vi "EncoderForward.vi"(8 "EncoderDevRef 4":T2={"DevStatus"={"status"=FALSE, "code"=0, "source"=""}, "EncoderIndex"=enum."Invalid", "CounterIndex"=enum."Ctr 1", "DistancePerCount"=2.0, "Decoding Type"=enum."4x"}, 9 "RobotDriveDevRef":T6={"DevStatus"={"status"=FALSE, "code"=0, "source"=""}, "Motors[]"=[], "Square Inputs"=FALSE, "Max Output"=1.0, "Isochronous"=FALSE}, 10 "EncoderDevRef":T2={"DevStatus"={"status"=FALSE, "code"=0, "source"=""}, "EncoderIndex"=enum."Invalid", "CounterIndex"=enum."Ctr 1", "DistancePerCount"=2.0, "Decoding Type"=enum."4x"}, 11 "Target":dbl format="%#_13g") -> (0 "EncoderDevRef 3":T2={"DevStatus"={"status"=FALSE, "code"=0, "source"=""}, "EncoderIndex"=enum."Invalid", "CounterIndex"=enum."Ctr 1", "DistancePerCount"=2.0, "Decoding Type"=enum."4x"}, 1 "RobotDriveDevRef 2":T6={"DevStatus"={"status"=FALSE, "code"=0, "source"=""}, "Motors[]"=[], "Square Inputs"=FALSE, "Max Output"=1.0, "Isochronous"=FALSE}, 2 "EncoderDevRef 2":T2={"DevStatus"={"status"=FALSE, "code"=0, "source"=""}, "EncoderIndex"=enum."Invalid", "CounterIndex"=enum."Ctr 1", "DistancePerCount"=2.0, "Decoding Type"=enum."4x"})   [LabVIEW 2013]
uses:
  <vilib>/Rock Robotics/WPI/RobotDrive/WPI_RobotDriveDevRef.ctl
  <vilib>/Rock Robotics/WPI/MotorControl/WPI_MotorControlDeviceRef.ctl
  <vilib>/Rock Robotics/SystemInterfaces/Typedef/FPGA_TypedefDigitalModule.ctl
  <vilib>/Rock Robotics/SystemInterfaces/DIO/FPGA_DIOPWMChannel.ctl
  <vilib>/Rock Robotics/WPI/PWM/WPI_PWMDeadband.ctl
  <vilib>/Rock Robotics/WPI/CAN/Jaguar/SubVIs/WPI_CANJaguar_ControlMode.ctl
  <vilib>/Rock Robotics/WPI/PWM/WPI_PWMTransform_ConPane.ctl
  <vilib>/Rock Robotics/WPI/Encoder/WPI_EncoderDevRef.ctl
  <vilib>/Rock Robotics/SystemInterfaces/Encoder/FPGA_EncoderIdx.ctl
  <vilib>/Rock Robotics/SystemInterfaces/Counter/FPGA_CounterCtrSystemIndex.ctl
  <vilib>/Rock Robotics/WPI/Encoder/WPI_EncoderType.ctl
  <vilib>/addons/control/pid/pid.llb/PID (DBL).vi
  <vilib>/addons/control/pid/NI_PID_pid.lvlib
panel:
  out "dt out (s)":dbl format="%.3f"
  out "Right Distance":dbl(graph)
  out "Right Motor Power":dbl(graph)
  out "Left Motor Power":dbl(graph)
  out "Left Distance":dbl(graph)
  in  "PID gains 3":T1={"proportional gain (Kc)"=0.15, "integral time (Ti, min)"=0.0, "derivative time (Td, min)"=0.0}
  in  "output range 3":cluster{"output high":dbl, "output low":dbl}={"output high"=1.0, "output low"=-1.0}
  in  "output range 2":cluster{"output high":dbl, "output low":dbl}={"output high"=1.0, "output low"=-1.0}
  in  "PID gains 2":T1={"proportional gain (Kc)"=0.15, "integral time (Ti, min)"=0.0, "derivative time (Td, min)"=0.0}
  # "Stop?"
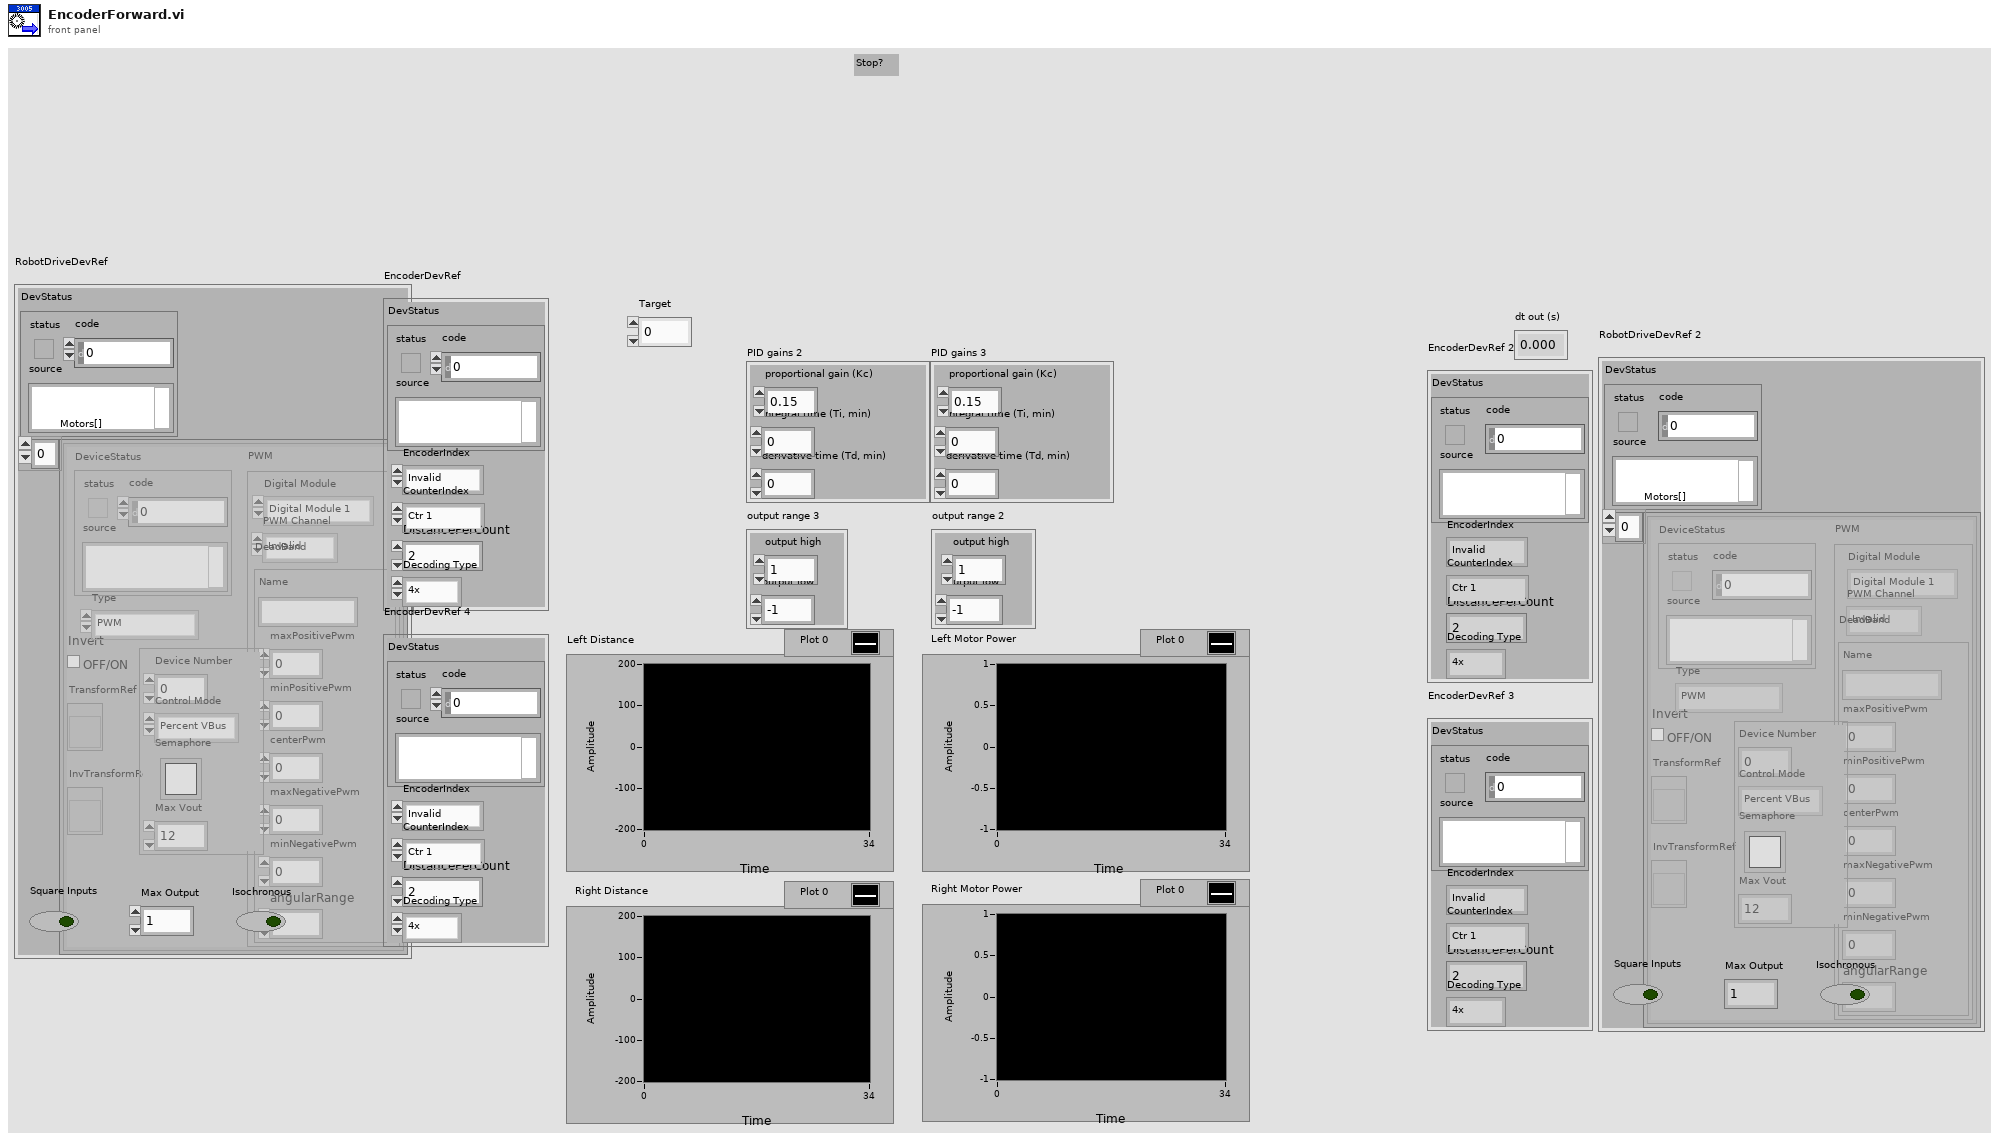
[diagram p1: front panel]
types:
  T1 = cluster{"proportional gain (Kc)":dbl, "integral time (Ti, min)":dbl, "derivative time (Td, min)":dbl}
  T2 = typedef "WPI_EncoderDevRef.ctl" = cluster{"DevStatus":errorcluster, "EncoderIndex":T3, "CounterIndex":T4, "DistancePerCount":dbl, "Decoding Type":T5}
  T3 = typedef "FPGA_EncoderIdx.ctl" = enum8{"Enc 0", "Enc 1", "Enc 2", "Enc 3", "Invalid"}
  T4 = typedef "FPGA_CounterCtrSystemIndex.ctl" = enum8{"Ctr 0", "Ctr 1", "Ctr 2", "Ctr 3", "Ctr 4", "Ctr 5", "Ctr 6", "Ctr 7", "Invalid"}
  T5 = typedef "WPI_EncoderType.ctl" = enum16{"1x", "2x", "4x"}
  T6 = typedef "WPI_RobotDriveDevRef.ctl" = cluster{"DevStatus":errorcluster, "Motors[]":T7[], "Square Inputs":bool, "Max Output":dbl, "Isochronous":bool}
  T7 = typedef "WPI_MotorControlDeviceRef.ctl" = cluster{"DeviceStatus":errorcluster, "Type":enum16{"PWM", "CAN"}, "PWM":cluster{"Digital Module":T8, "PWM Channel":T9, "DeadBand":T10}, "CAN":cluster{"Device Number":u8, "Control Mode":T11, "Semaphore":T12, "Max Vout":dbl}, "Invert":bool, "TransformRef":T13, "InvTransformRef":T13}
  T8 = typedef "FPGA_TypedefDigitalModule.ctl" = enum16{"Digital Module 1", "Digital Module 2"}
  T9 = typedef "FPGA_DIOPWMChannel.ctl" = enum8{"PWM 1", "PWM 2", "PWM 3", "PWM 4", "PWM 5", "PWM 6", "PWM 7", "PWM 8", "PWM 9", "PWM 10", "Invalid"}
  T10 = typedef "WPI_PWMDeadband.ctl" = cluster{"Name":string, "maxPositivePwm":i32, "minPositivePwm":i32, "centerPwm":i32, "maxNegativePwm":i32, "minNegativePwm":i32, "angularRange":u16}
  T11 = typedef "WPI_CANJaguar_ControlMode.ctl" = enum8{"Percent VBus", "Current", "Speed", "Position", "Voltage"}
  T12 = typedef "Semaphore RefNum" = refnum<k1>
  T13 = typedef "WPI_PWMTransform_ConPane.ctl" = refnum<vi>
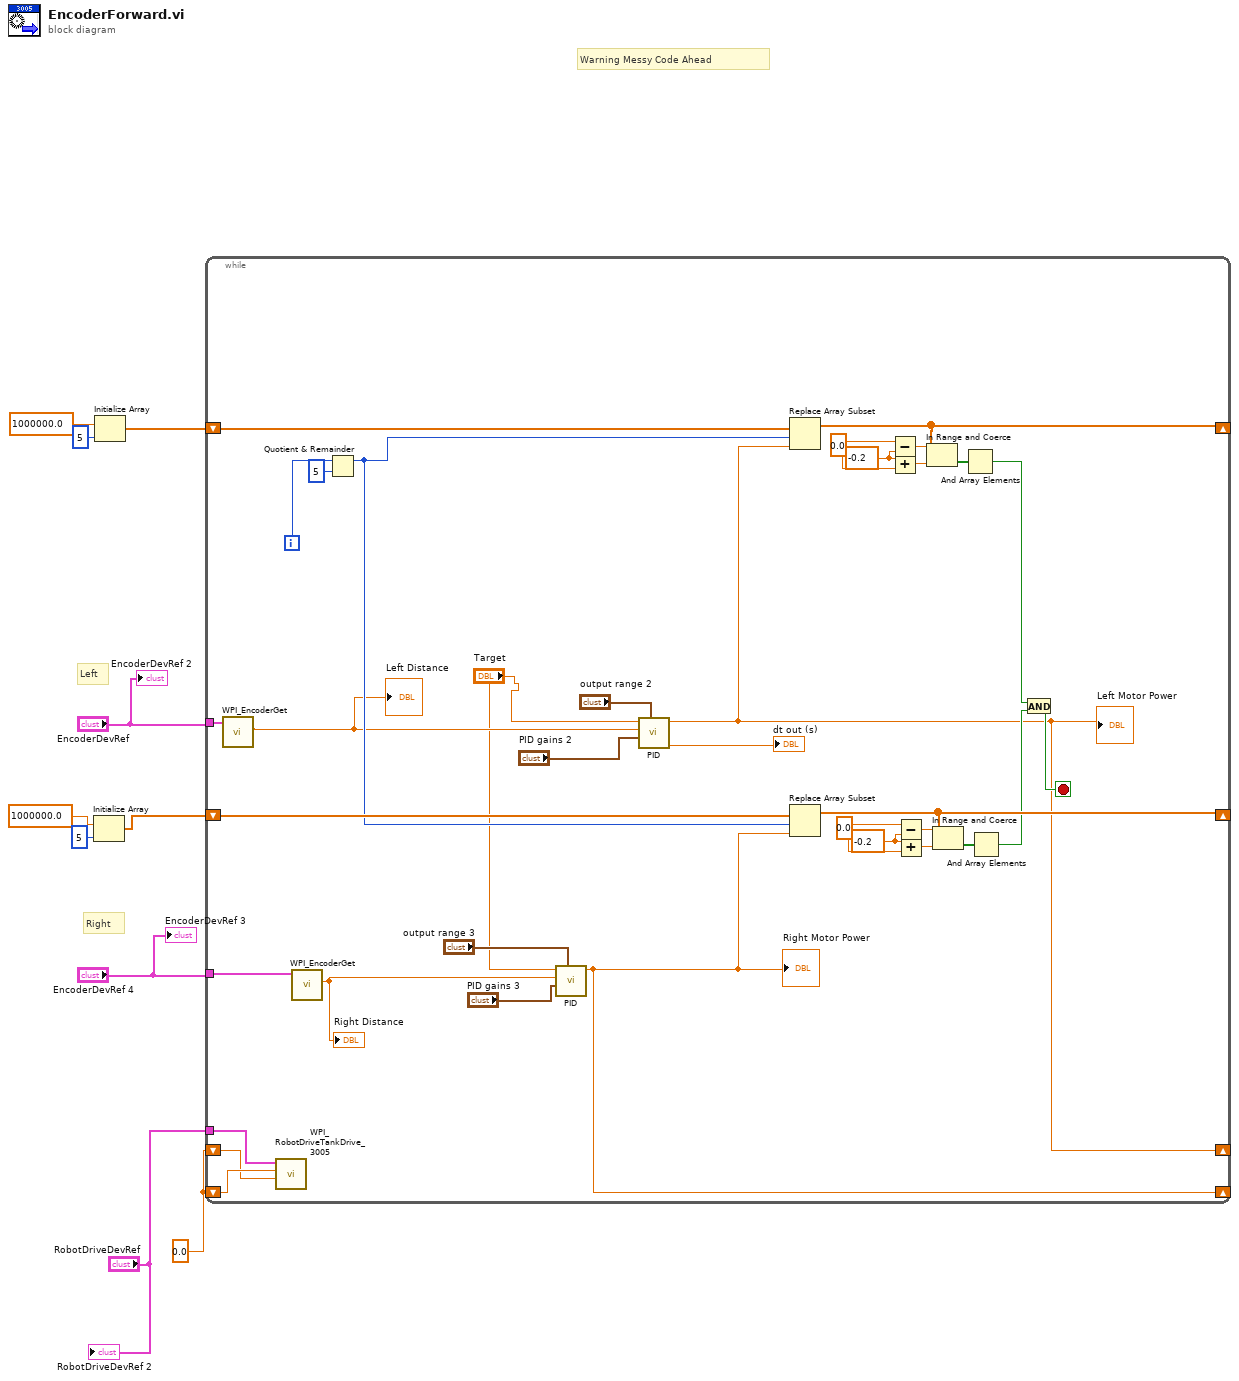
[diagram p0: block diagram]
diagram:
  w3 = 0.0 ("output")
  # "Warning Messy Code Ahead"
  # "Right"
  # "Left"
  n1 = Initialize Array(1000000.0 ("element"), 5 ("dimension size")) -> (w6:dbl[])
  n2 = Initialize Array(1000000.0 ("element"), 5 ("dimension size")) -> (w7:dbl[])
  n3 = while {
    shift-right: [w18] -> _
    shift-left: w3 -> [w28]
    tunnel: "RobotDriveDevRef" -> [w44]
    shift-right: [w12] -> _
    shift-left: w7 -> [w42]
    tunnel: "EncoderDevRef" -> [w40]
    shift-right: [w37] -> _
    shift-left: w6 -> [w34]
    tunnel: "EncoderDevRef 4" -> [w39]
    shift-right: [w21] -> _
    shift-left: w3 -> [w29]
    i -> [w41]
    stop <- w32 stop-if-true
    w13 = -0.2 ("x")
    w14 = 0.0 ("x")
    w19 = -0.2 ("x")
    w20 = 0.0 ("x")
    n4 = call <vilib>:"WPI_EncoderGet.vi"("EncoderDevRef"=w40) -> ("Distance"=w25:dbl)  [unwired: 1 in, 9 out]
    "Left Distance" <- w25
    n5 = call <vilib>:"WPI_RobotDriveTankDrive_3005.vi"("Right axis value"=w28, "Left axis value"=w29, "RobotDriveDevRef"=w44) -> ()  [unwired: 6 in, 3 out]
    n6 = call <vilib>:"WPI_EncoderGet.vi"("EncoderDevRef"=w39) -> ("Distance"=w26:dbl)  [unwired: 1 in, 9 out]
    "Right Distance" <- w26
    n7 = Quotient & Remainder(x=w41, y=5) -> (x-y*floor(x/y)=w30:i32)  [unwired: 1 out]
    n8 = call-poly <vilib>:"PID.vi"("output range"="output range 3", "PID gains"="PID gains 3", "process variable"=w26, "setpoint"="Target") -> ("output"=w21:dbl)  [unwired: 6 in, 1 out]
    "Right Motor Power" <- w21
    n9 = call-poly <vilib>:"PID.vi"("output range"="output range 2", "PID gains"="PID gains 2", "process variable"=w25, "setpoint"="Target") -> ("dt out (s)"=→"dt out (s)":dbl, "output"=w18:dbl)  [unwired: 6 in]
    "Left Motor Power" <- w18
    n10 = Replace Array Subset(array=w42, new element=w18, index=w30) -> (w12:dbl[])
    n11 = Replace Array Subset(array=w34, new element=w21, index=w30) -> (w37:dbl[])
    n12 = Subtract(x=w14, y=w13) -> (x-y=w15:dbl)
    n13 = Add(x=w13, y=w14) -> (x+y=w17:dbl)
    n14 = Subtract(x=w20, y=w19) -> (x-y=w35:dbl)
    n15 = Add(x=w19, y=w20) -> (x+y=w38:dbl)
    n16 = In Range and Coerce(upper limit=w15, x=w12, lower limit=w17) -> (In Range?=w16:bool[])  [unwired: 1 out]
    n17 = In Range and Coerce(upper limit=w35, x=w37, lower limit=w38) -> (In Range?=w36:bool[])  [unwired: 1 out]
    n18 = And Array Elements(Boolean array=w16) -> (logical AND=w11:bool)
    n19 = And Array Elements(Boolean array=w36) -> (logical AND=w31:bool)
    n20 = And(x=w11, y=w31) -> (x .and. y?=w32:bool)
  }
  "RobotDriveDevRef 2" <- "RobotDriveDevRef"
  "EncoderDevRef 2" <- "EncoderDevRef"
  "EncoderDevRef 3" <- "EncoderDevRef 4"
